vi "Assert Log File Is Valid.vi"(7 "Error":i32=5, 8 "error in (no error)":errorcluster, 11 "Embedded Data Logger System Tests in":refnum<class "Embedded Data Logger System Tests.lvclass">) -> (0 "error out":errorcluster, 3 "Embedded Data Logger System Tests out":refnum<class "Embedded Data Logger System Tests.lvclass">)   [LabVIEW 2018, in "Embedded Data Logger System Tests.lvclass"]
uses:
  Embedded Data Logger System Tests.lvclass
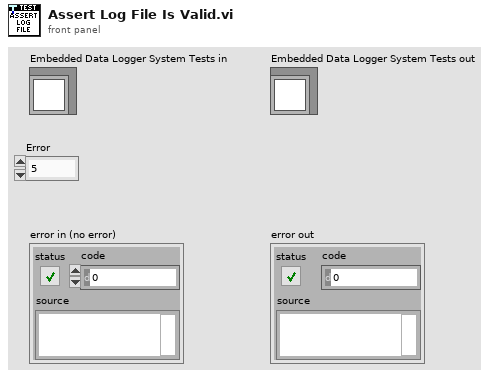
[diagram p1: front panel]
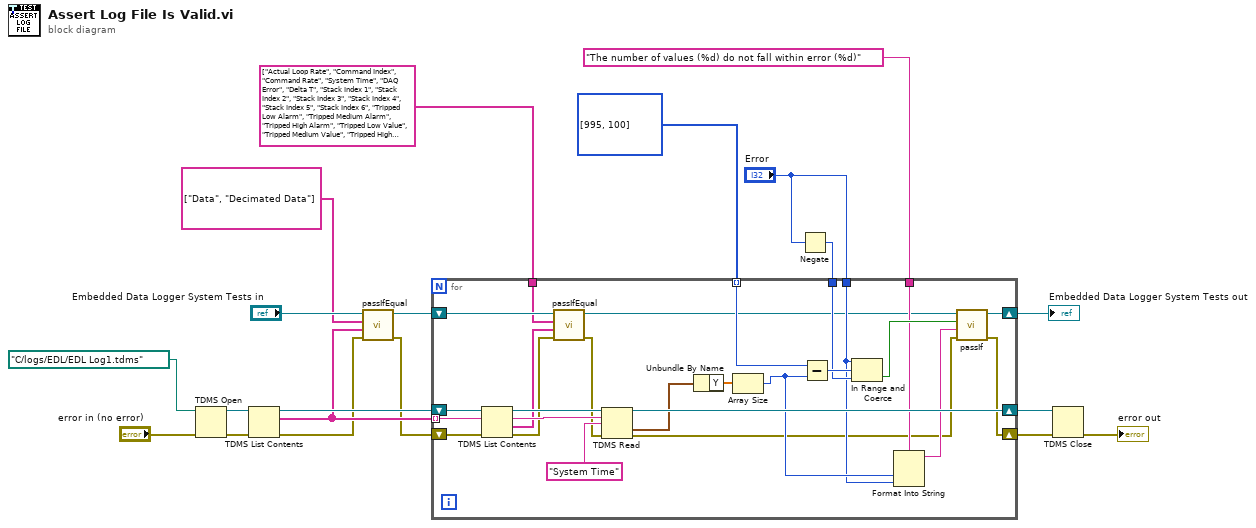
[diagram p0: block diagram]
diagram:
  n1 = TDMS Open(8:"error in (no error)", 11:path "C:/logs/EDL/EDL Log1.tdms" ("file path")) -> (0:w16:errorcluster, 3:w17:refnum<k34>)  [unwired: 5 in]
  n2 = TDMS List Contents(4:w16, 7:w17) -> (0:w3:errorcluster, 2:w4:string[], 3:w14:refnum<k34>)  [unwired: 1 in, 1 out]
  n3 = call-dynamic "passIfEqual.vi"("error in (no error)"=w3, "y"=w4, "x"=string[] ["Data", "Decimated Data"] ("group names"), "TestCase in"="Embedded Data Logger System Tests in") -> ("error out"=w2:errorcluster, "TestCase out"=w6:refnum<class "Embedded Data Logger System Tests.lvclass">)  [unwired: 6 in]
  n4 = Negate(x="Error") -> (-x=w8:i32)
  n5 = for {
    shift-right: [w31] -> w15
    shift-left: w2 -> [w30]
    shift-right: [w46] -> w13
    shift-left: w14 -> [w29]
    tunnel: w4 -> [w27] mode=indexing
    shift-right: [w42] -> w11
    shift-left: w6 -> [w44]
    tunnel: i32[] [995, 100] -> [w40] mode=indexing
    tunnel: "Error" -> [w34]
    tunnel: w8 -> [w38]
    tunnel: "The number of values (%d) do not fall within error (%d)" ("message (\"\")") -> [w35]
    tunnel: string[] ["Actual Loop Rate", "Command Index", "Command Rate", "System Time", "DAQ Error", "Delta T", "Stack Index 1", "Stack Index 2", "Stack Index 3", "Stack Index 4", "Stack Index 5", "Stack Index 6", "Tripped Low Alarm", "Tripped Medium Alarm", "Tripped High Alarm", "Tripped Low Value", "Tripped Medium Value", "Tripped High Value", "RT Engine Build", "HP Loop Duration", "LP Loop Duration", "System Command", "Streamed Channel Count", "Max Streamed Channels", "Model Count", "Maximum GENs", "Generator Engine State", "Watchdog Timer", "HS TCP Overflow Count", "Host IP", "Trace Enabled Flag", "Detailed Tracing Flag", "VI Tracing Flag", "Trace Buffer Size", "Thread Tracing Flag", "Absolute Time", "System Time - Microseconds", "ASAM XIL EESPort Trigger", "ASAM XIL EESPort Trigger Count", "Failure Count", "Analysis State", "TCP Data Packet Loss", "WPL Overflow Count", "WPL TCP Overflow Count", "WPL Error Count", "WPL Error Code", "Streamed Waveform Count", "Iteration", "Last Late Iteration", "Real-Time Sequence Command", "Real-Time Sequence Count", "HP Loop Wakeup Status", "HP-LP Overwrite", "LP Data Count", "HP Count", "LP Count", "Log Status"] ("channel names") -> [w24]
    n6 = TDMS List Contents(4:w30, 6:w27, 7:w29) -> (0:w22:errorcluster, 1:w23:string[], 2:w26:string, 3:w28:refnum<k34>)
    n7 = call-dynamic "passIfEqual.vi"("error in (no error)"=w22, "y"=w23, "x"=w24, "TestCase in"=w44) -> ("error out"=w21:errorcluster, "TestCase out"=w25:refnum<class "Embedded Data Logger System Tests.lvclass">)  [unwired: 6 in]
    n8 = TDMS Read(0:w28, 5:w26, 7:"System Time", 11:w21) -> (4:w46:refnum<k34>, 10:w43:waveform(dbl), 15:w32:errorcluster)  [unwired: 4 in, 3 out]
    n9 = Unbundle By Name(w43) -> ("Y"=w41:dbl[])
    n10 = Array Size(array=w41) -> (size(s)=w36:i32)
    n11 = Subtract(x=w40, y=w36) -> (x-y=w39:i32)
    n12 = In Range and Coerce(upper limit=w34, x=w39, lower limit=w38) -> (In Range?=w37:bool)  [unwired: 1 out]
    n13 = Format Into String(format string=w35, w36, w34) -> (resulting string=w33:string)  [unwired: 2 in, 1 out]
    n14 = call-dynamic "passIf.vi"("error in (no error)"=w32, "message (\"\")"=w33, "pass"=w37, "TestCase in"=w25) -> ("error out"=w31:errorcluster, "TestCase out"=w42:refnum<class "Embedded Data Logger System Tests.lvclass">)  [unwired: 6 in]
  }
  "Embedded Data Logger System Tests out" <- w11
  n15 = TDMS Close(8:w15, 11:w13) -> (0:→"error out":errorcluster)  [unwired: 1 out]
